vi "ArmJoystickControl.vi"(1 "Joystick control":T2) -> (0 "ArmTargetPointCommand":T1)   [LabVIEW 2017]
uses:
  TypeDefs/JoystickControls.ctl
  TypeDefs/ArmTargetPointCommand.ctl
panel:
  in  "Grab position":bool
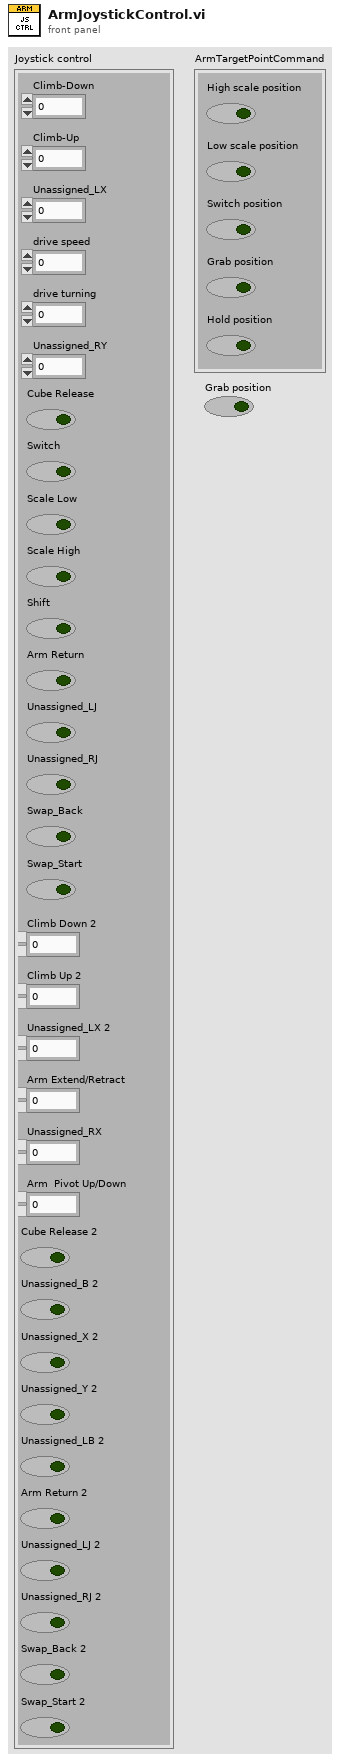
[diagram p1: front panel]
types:
  T1 = typedef "ArmTargetPointCommand.ctl" = cluster{"Hold position":bool, "High scale position":bool, "Low scale position":bool, "Switch position":bool, "Grab position":bool}
  T2 = typedef "JoystickControls.ctl" = cluster{"drive speed":dbl, "drive turning":dbl, "Unassigned_LX":dbl, "Unassigned_RY":dbl, "Cube Release":bool, "Climb-Up":dbl, "Climb-Down ":dbl, "Switch":bool, "Scale Low":bool, "Scale High":bool, "Shift":bool, "Arm Return":bool, "Unassigned_LJ":bool, "Unassigned_RJ":bool, "Swap_Back":bool, "Swap_Start":bool, "Arm Extend/Retract":dbl, "Unassigned_RX":dbl, "Unassigned_LX 2":dbl, "Arm  Pivot Up/Down ":dbl, "Cube Release 2":bool, "Climb Up 2":dbl, "Climb Down 2":dbl, "Unassigned_B 2":bool, "Unassigned_X 2":bool, "Unassigned_Y 2":bool, "Unassigned_LB 2":bool, "Arm Return 2":bool, "Unassigned_LJ 2":bool, "Unassigned_RJ 2":bool, "Swap_Back 2":bool, "Swap_Start 2":bool}
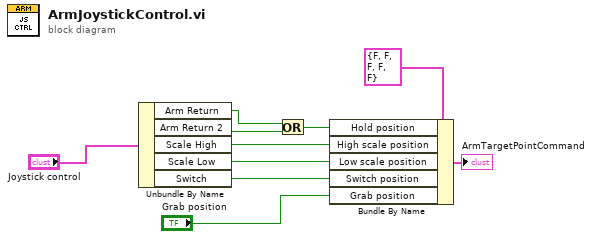
[diagram p0: block diagram]
diagram:
  n1 = Unbundle By Name("Joystick control") -> ("Arm Return"=w4:bool, "Arm Return 2"=w3:bool, "Scale High"=w5:bool, "Scale Low"=w6:bool, "Switch"=w7:bool)
  n2 = Or(x=w4, y=w3) -> (x .or. y?=w2:bool)
  n3 = Bundle By Name(cluster=T1 {"Hold position"=FALSE, "High scale position"=FALSE, "Low scale position"=FALSE, "Switch position"=FALSE, "Grab position"=FALSE} ("ArmTargetPointCommand"), "Hold position"=w2, "High scale position"=w5, "Low scale position"=w6, "Switch position"=w7, "Grab position"="Grab position") -> (→"ArmTargetPointCommand":T1)
